vi "Assignment.vi"() -> ()   [LabVIEW 2021]
doc: "https://icons8.com/icon/85465/time\nhttps://icons8.com/icon/44369/cheap-2\nhttps://icons8.com/icon/44372/expensive-price\nhttps://icons8.com/icon/17077/info-squared"
uses:
  Resources/Enum.ctl
  <vilib>/Utility/error.llb/DialogType.ctl
  <vilib>/Utility/file.llb/Write Delimited Spreadsheet (string).vi
panel:
  in  "infoTab":enum32{"InfoTab"}(tab)
  in  "btnInfo":bool
  out "Message":string
  out "isDeluxe":bool
  out "Time Left":dbl(slide) scale=0.0..5.0
  in  "Air Dry \nPosition Switch":bool
  in  "Main Wash \nPosition Switch":bool
  in  "Under Body \nWash Position \nSwitch":bool
  out "Vehicle Out Of Position":bool
  out "Air Dry":bool
  out "Clear Water Rinse":bool
  out "Main High Pressure Wash":bool
  out "Soap Application":bool
  out "Under Body Wash":bool
  in  "btnStop":bool
  in  "btnEconomy":bool
  in  "btnDeluxe":bool
  # "Please select Car Wash Mode"
  # "Deluxe Wash"
  # "Economy Wash"
  # "Message"
  # "Deluxe Wash:\n1. Under Body Wash\n2. Main Car Wash\n3. Air Dry Cycle"
  # "Economy Wash:"
  # "1. Main Car Wash"
  # "approx 25 seconds"
  # "approx 15 seconds"
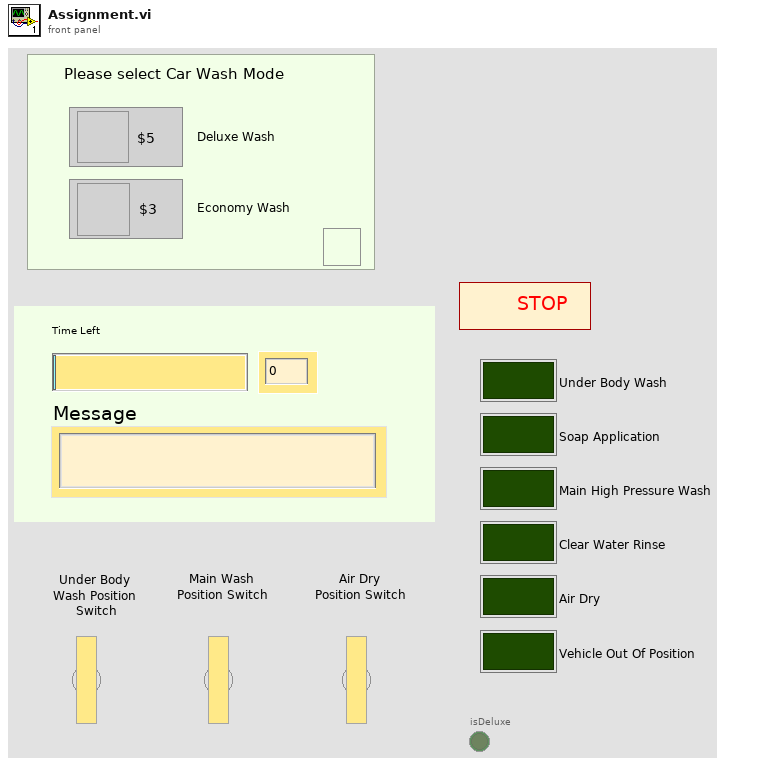
[diagram p1: front panel]
types:
  T1 = typedef "Enum.ctl" = enum16{"Start", "SelectMode", "UnderBodyTimer", "UnderBody", "Soap Timer", "Soap", "MainWashTimer", "MainWash", "RinseTimer", "Rinse", "AirDryTimer", "AirDry", "Trasmit", "End"}
  T2 = enum8{"Enabled", "Disabled", "Disabled and Grayed Out"}
  T3 = typedef "DialogType.ctl" = u16
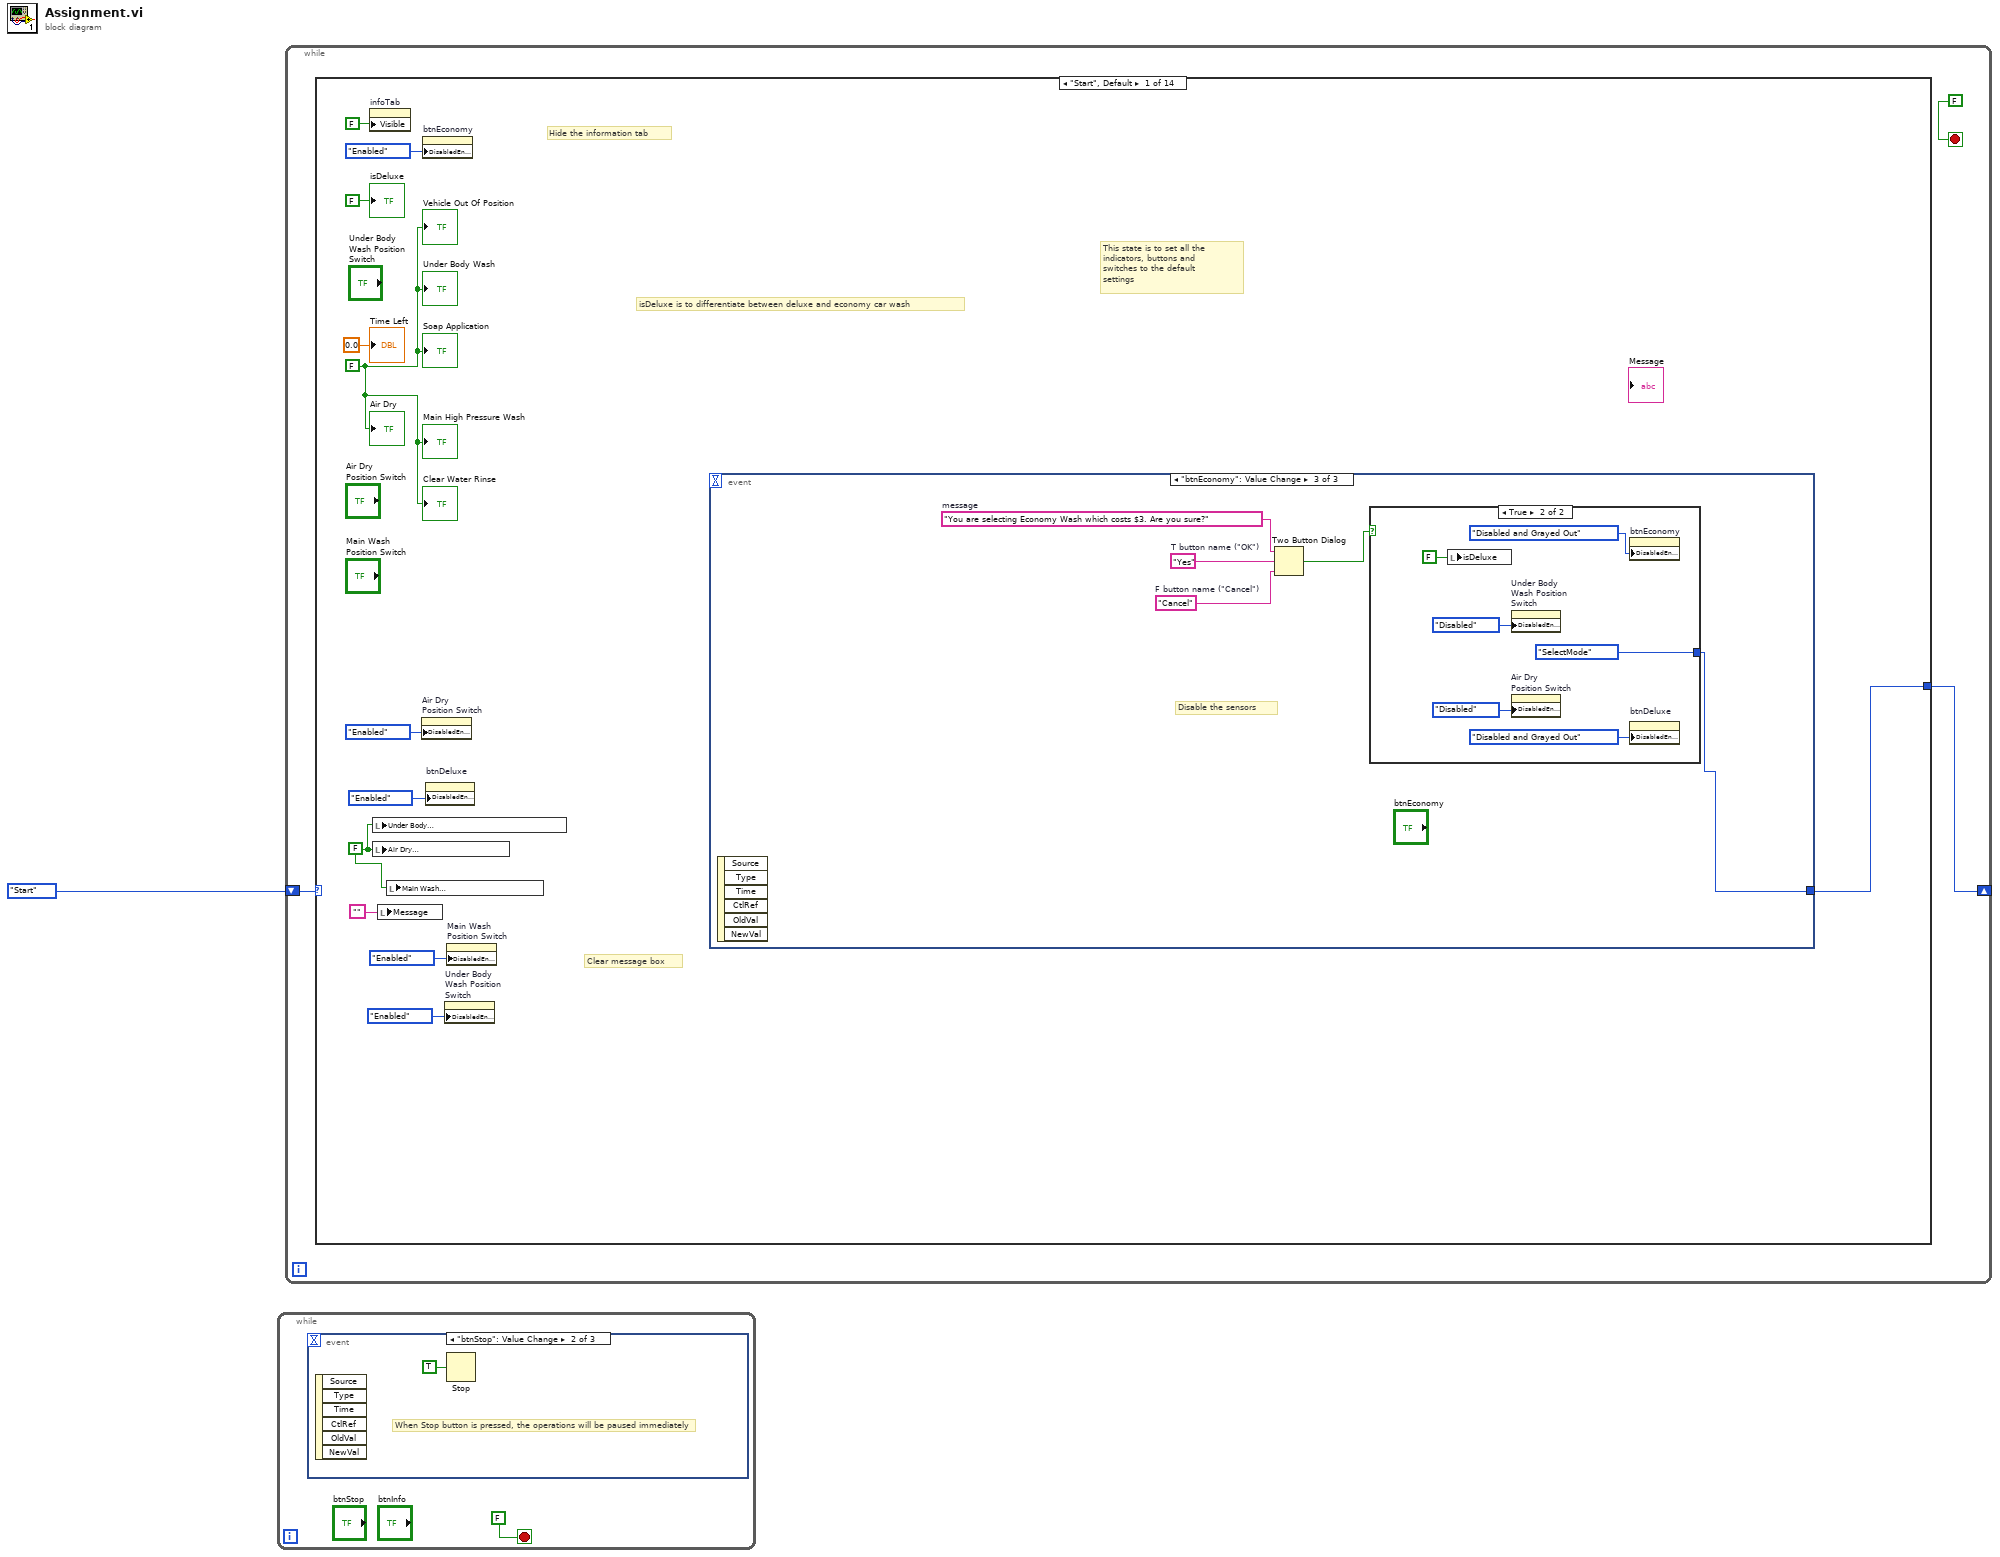
[diagram p0: block diagram]
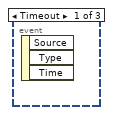
[diagram p2: hidden frame]
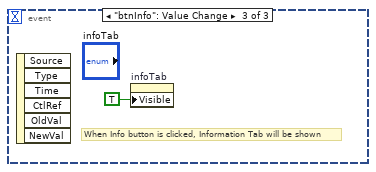
[diagram p3: hidden frame]
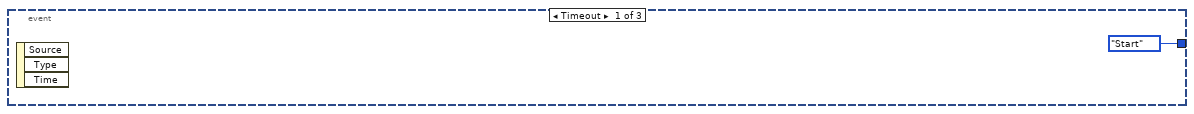
[diagram p4: hidden frame]
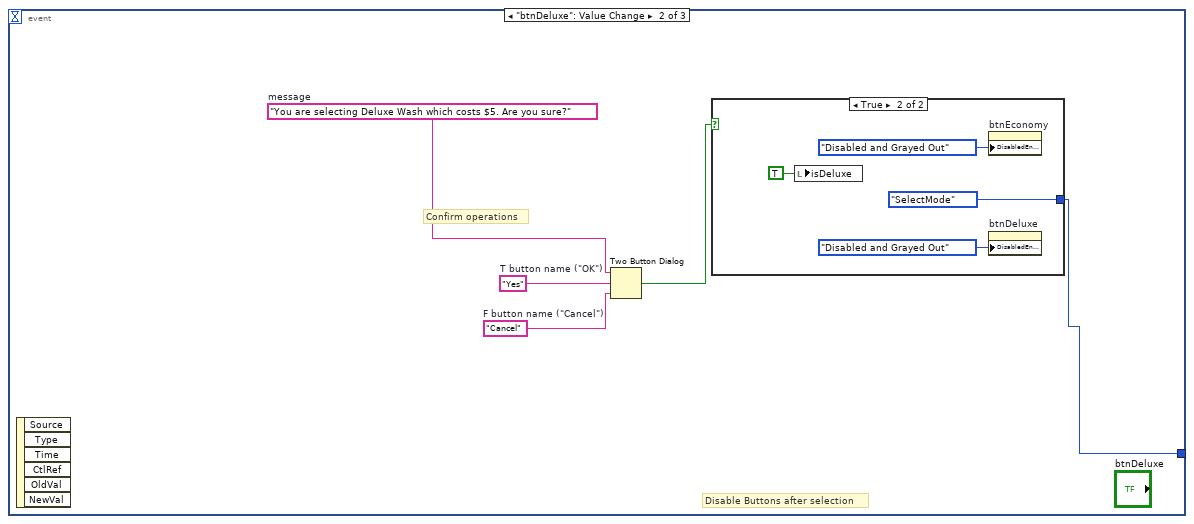
[diagram p5: hidden frame]
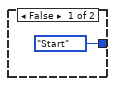
[diagram p6: hidden frame]
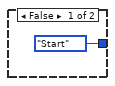
[diagram p7: hidden frame]
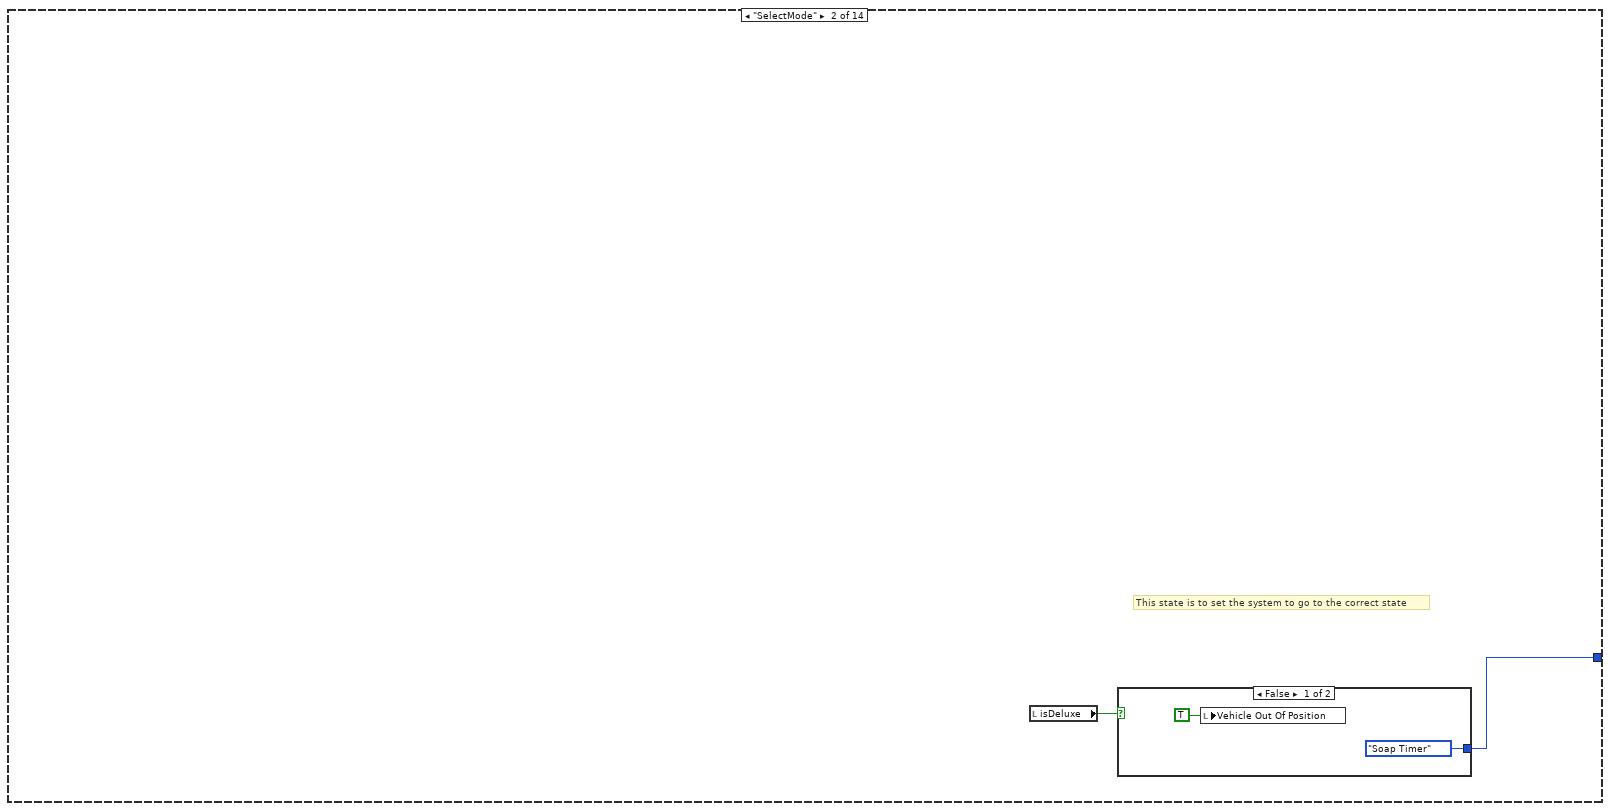
[diagram p8: hidden frame]
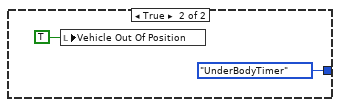
[diagram p9: hidden frame]
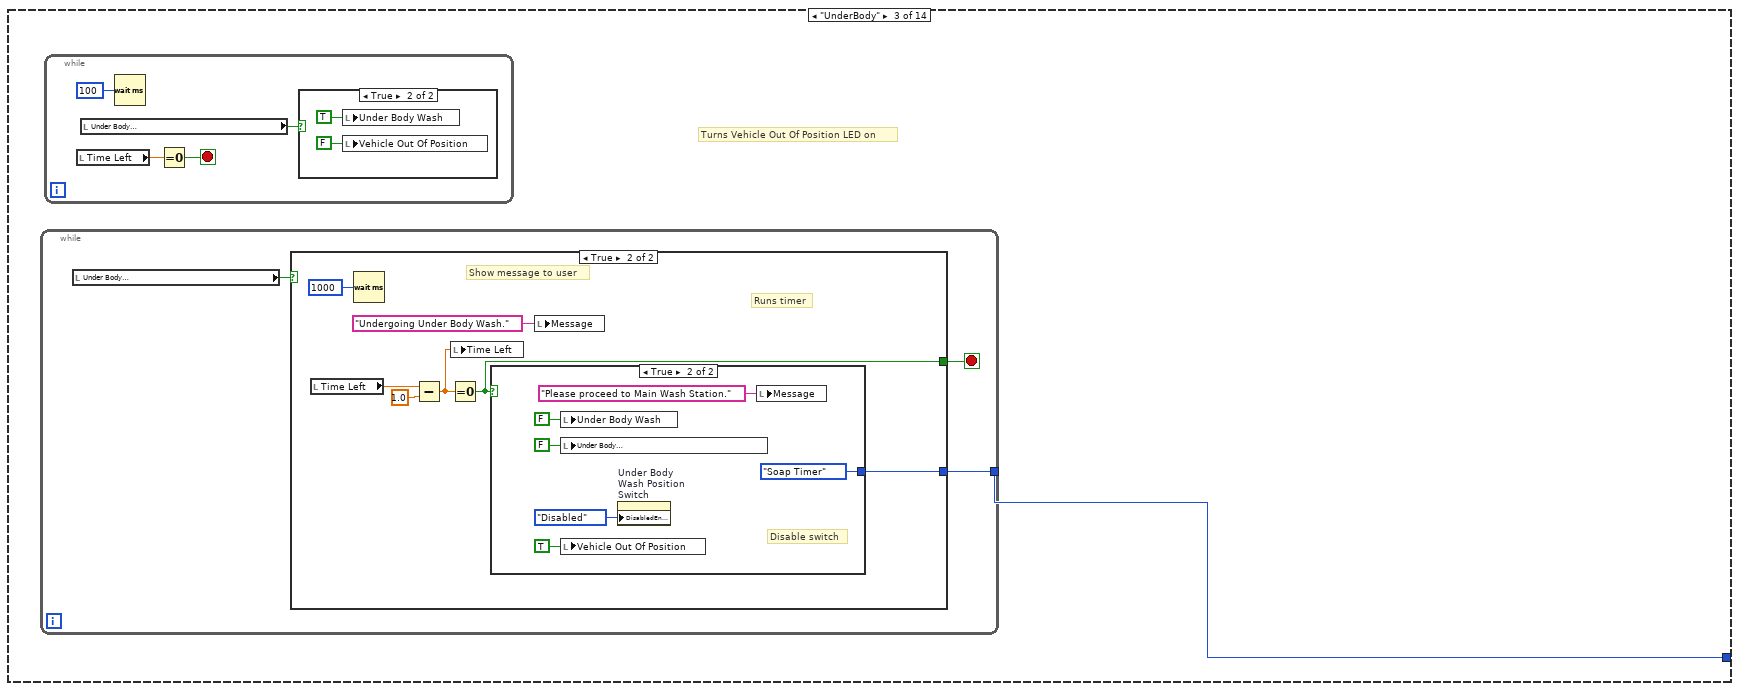
[diagram p10: hidden frame]
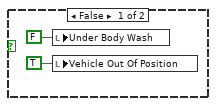
[diagram p11: hidden frame]
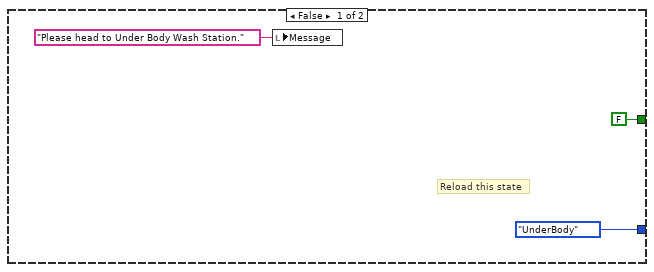
[diagram p12: hidden frame]
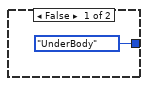
[diagram p13: hidden frame]
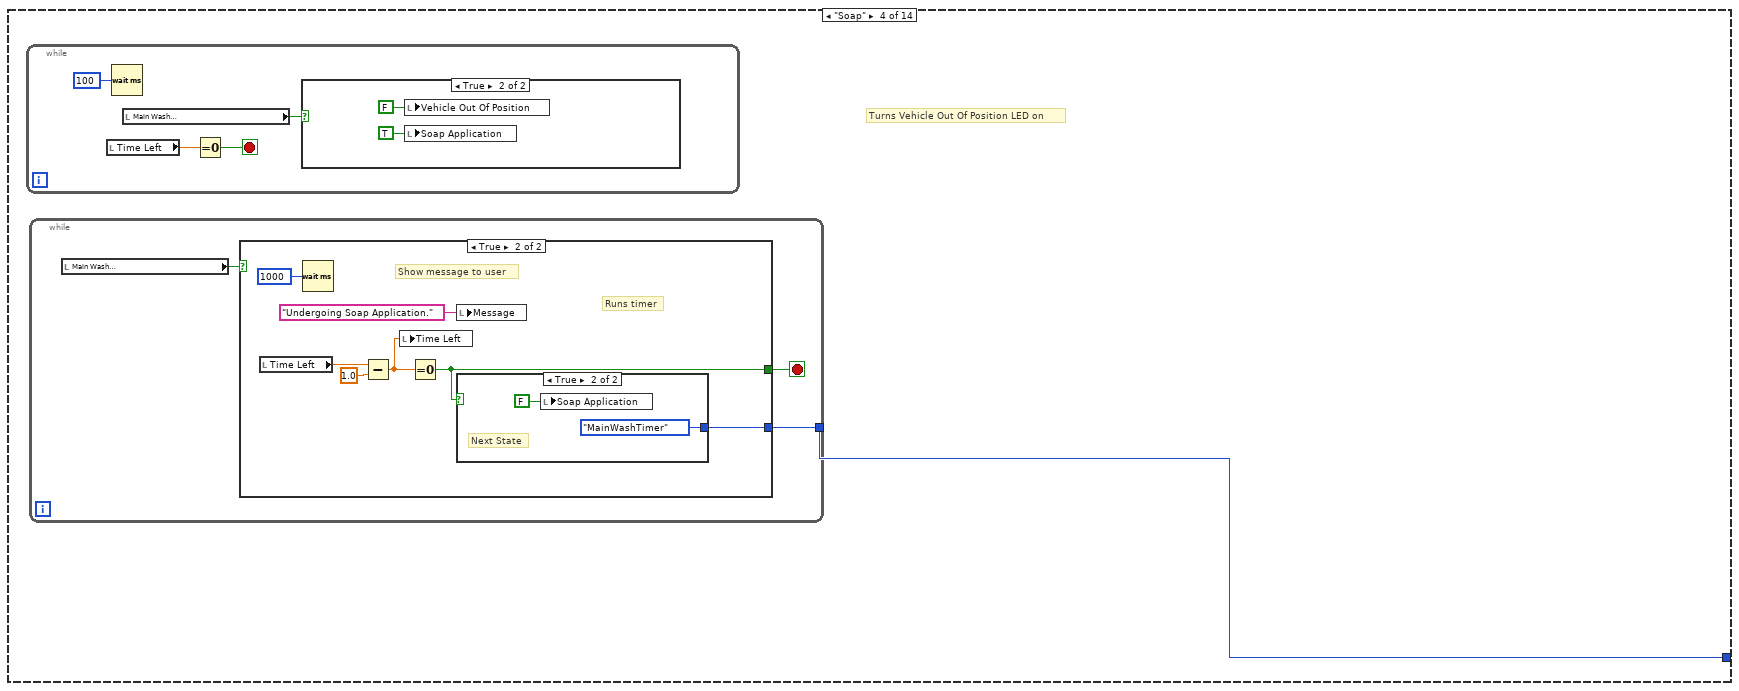
[diagram p14: hidden frame]
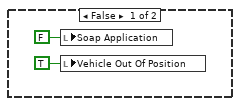
[diagram p15: hidden frame]
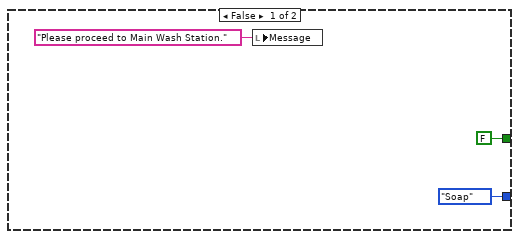
[diagram p16: hidden frame]
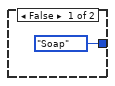
[diagram p17: hidden frame]
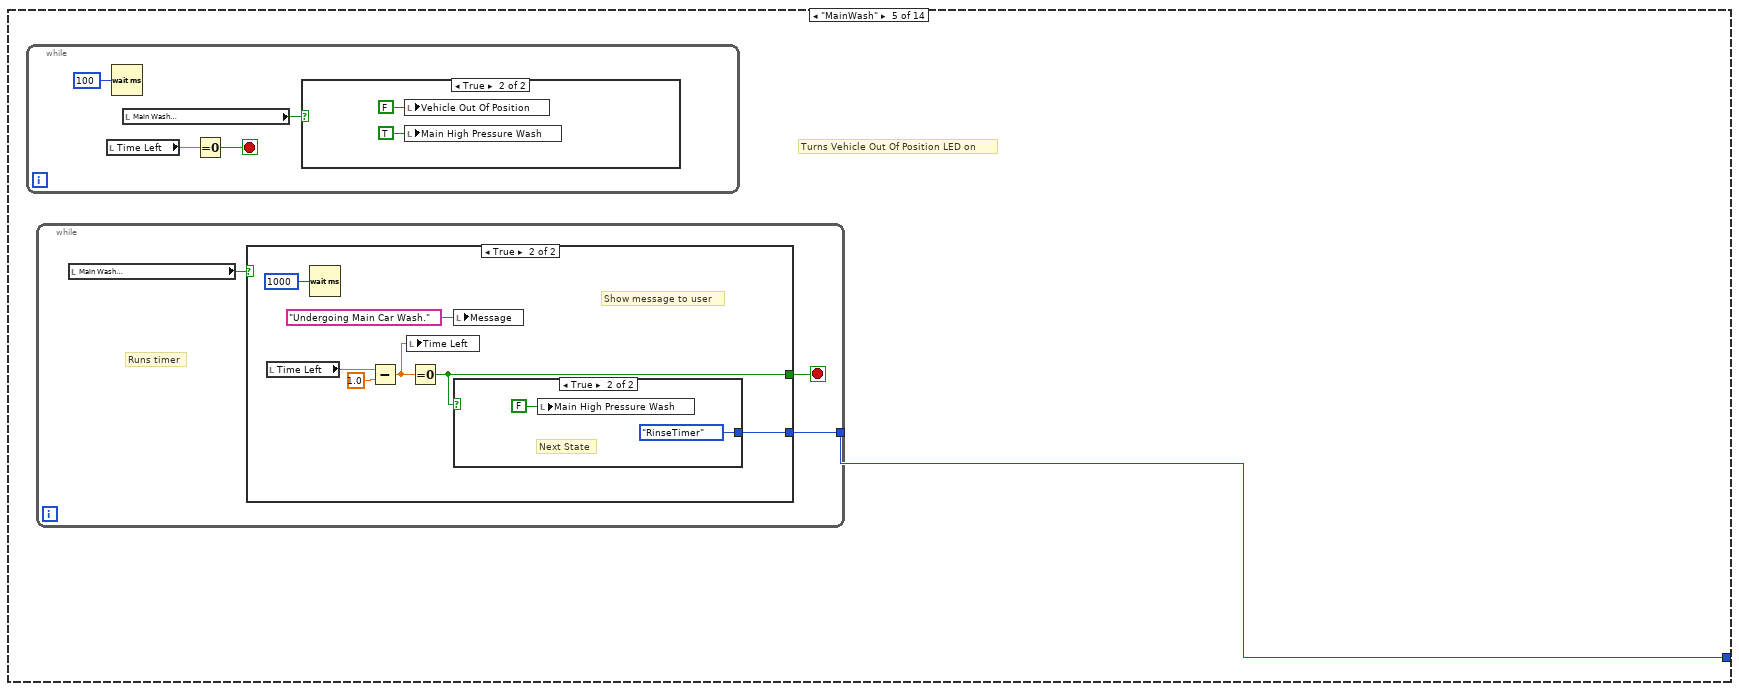
[diagram p18: hidden frame]
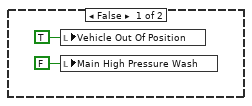
[diagram p19: hidden frame]
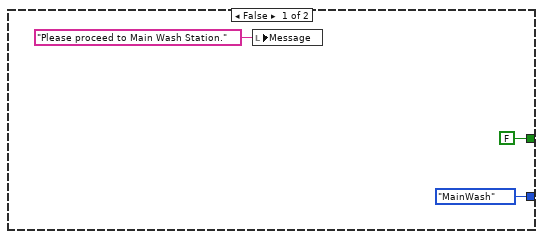
[diagram p20: hidden frame]
diagram:
  n1 = while {
    stop <- FALSE stop-if-true
    n2 = event shown="[1] \"btnStop\": Value Change" {
      selector: _ -> [_ _ _]
      dyn-events: _ -> [_ _ _]
      timeout: _ -> [_ _ _]
      event Timeout {
        n3 = event-data() -> ()  [unwired: 1 in, 3 out]
      }
      event "btnStop": Value Change {
        # "When Stop button is pressed, the operations will be paused immediately"
        n4 = event-data() -> ()  [unwired: 1 in, 6 out]
        n5 = Stop(stop? (T)=TRUE) -> ()
      }
      event "btnInfo": Value Change {
        # "When Info button is clicked, Information Tab will be shown"
        n6 = event-data() -> ()  [unwired: 1 in, 6 out]
        n7 = property on="infoTab" class="TabCtl (strict)"("Visible"=TRUE) -> ()  [unwired: 2 in, 2 out]
      }
    }
  }
  n8 = while {
    shift-right: [w6] -> _
    shift-left: Enum."Start" -> [w7]
    stop <- FALSE stop-if-true
    n9 = case shown="\"Start\", Default" w7 {
      tunnel: [w19 w43 w49 w78 w103 w129 w162 Enum."End" Enum."Start" Enum."UnderBody" Enum."Soap" Enum."MainWash" Enum."Rinse" Enum."AirDry"] -> w6
      frame "Start", Default {
        w8 = FALSE ("Vehicle Out Of Positon")
        w18 = FALSE ("Air Dry \nPosition Switch")
        # "Clear message box"
        # "isDeluxe is to differentiate between deluxe and economy car wash"
        # "Hide the information tab"
        # "This state is to set all the indicators, buttons and switches to the default settings"
        n10 = property on="infoTab" class="TabCtl (strict)"("Visible"=FALSE) -> ()  [unwired: 2 in, 2 out]
        n11 = local write "Under Body \nWash Position \nSwitch"(w18) -> ()
        n12 = local write "Air Dry \nPosition Switch"(w18) -> ()
        n13 = local write "Message"("") -> ()
        n14 = local write "Main Wash \nPosition Switch"(w18) -> ()
        n15 = property on="Air Dry \nPosition Switch" class="Bool (strict)"("DisabledEnum"=T2."Enabled" ("Disabled")) -> ()  [unwired: 2 in, 2 out]
        n16 = property on="btnEconomy" class="Bool"("DisabledEnum"=T2."Enabled" ("Disabled")) -> ()  [unwired: 2 in, 2 out]
        n17 = property on="btnDeluxe" class="Bool"("DisabledEnum"=T2."Enabled" ("Disabled")) -> ()  [unwired: 2 in, 2 out]
        n18 = property on="Under Body \nWash Position \nSwitch" class="Bool (strict)"("DisabledEnum"=T2."Enabled" ("Disabled")) -> ()  [unwired: 2 in, 2 out]
        n19 = property on="Main Wash \nPosition Switch" class="Bool (strict)"("DisabledEnum"=T2."Enabled" ("Disabled")) -> ()  [unwired: 2 in, 2 out]
        n20 = event shown="[2] \"btnEconomy\": Value Change" {
          selector: _ -> [_ _ _]
          dyn-events: _ -> [_ _ _]
          timeout: _ -> [_ _ _]
          tunnel: [Enum."Start" w21 w31] -> w19
          event Timeout {
            n21 = event-data() -> ()  [unwired: 1 in, 3 out]
          }
          event "btnDeluxe": Value Change {
            w23 = "You are selecting Deluxe Wash which costs $5. Are you sure?"  # message
            w24 = "Cancel"  # F button name ("Cancel")
            w25 = "Yes"  # T button name ("OK")
            # "Disable Buttons after selection"
            # "Confirm operations"
            n22 = event-data() -> ()  [unwired: 1 in, 6 out]
            n23 = Two Button Dialog(message=w23, 1:w24, 2:w25) -> (T button?=w22:bool)
            n24 = case shown="True" w22 {
              tunnel: [Enum."Start" ("f") Enum."SelectMode"] -> w21
              frame False {
              }
              frame True {
                n25 = local write "isDeluxe"(TRUE ("isDeluxe")) -> ()
                n26 = property on="btnEconomy" class="Bool"("DisabledEnum"=T2."Disabled and Grayed Out" ("Disabled")) -> ()  [unwired: 2 in, 2 out]
                n27 = property on="btnDeluxe" class="Bool"("DisabledEnum"=T2."Disabled and Grayed Out" ("Disabled")) -> ()  [unwired: 2 in, 2 out]
              }
            }
          }
          event "btnEconomy": Value Change {
            w32 = "You are selecting Economy Wash which costs $3. Are you sure?"  # message
            w34 = "Cancel"  # F button name ("Cancel")
            w33 = "Yes"  # T button name ("OK")
            # "Disable the sensors"
            n28 = event-data() -> ()  [unwired: 1 in, 6 out]
            n29 = Two Button Dialog(message=w32, 1:w34, 2:w33) -> (T button?=w35:bool)
            n30 = case shown="True" w35 {
              tunnel: [Enum."Start" ("f") Enum."SelectMode"] -> w31
              frame False {
              }
              frame True {
                n31 = local write "isDeluxe"(FALSE ("isDeluxe")) -> ()
                n32 = property on="Under Body \nWash Position \nSwitch" class="Bool (strict)"("DisabledEnum"=T2."Disabled" ("Disabled")) -> ()  [unwired: 2 in, 2 out]
                n33 = property on="Air Dry \nPosition Switch" class="Bool (strict)"("DisabledEnum"=T2."Disabled" ("Disabled")) -> ()  [unwired: 2 in, 2 out]
                n34 = property on="btnEconomy" class="Bool"("DisabledEnum"=T2."Disabled and Grayed Out" ("Disabled")) -> ()  [unwired: 2 in, 2 out]
                n35 = property on="btnDeluxe" class="Bool"("DisabledEnum"=T2."Disabled and Grayed Out" ("Disabled")) -> ()  [unwired: 2 in, 2 out]
              }
            }
          }
        }
        "isDeluxe" <- FALSE ("isDeluxe")
        "Time Left" <- 0.0 ("Time Left")
        "Main High Pressure Wash" <- w8
        "Clear Water Rinse" <- w8
        "Air Dry" <- w8
        "Under Body Wash" <- w8
        "Soap Application" <- w8
        "Vehicle Out Of Position" <- w8
      }
      frame "SelectMode" {
        # "This state is to set the system to go to the correct state"
        n36 = local read "isDeluxe"() -> (w44:bool)
        n37 = case shown="False" w44 {
          tunnel: [Enum."Soap Timer" Enum."UnderBodyTimer"] -> w43
          frame False {
            n38 = local write "Vehicle Out Of Position"(TRUE ("Vehicle Out Of Positon")) -> ()
          }
          frame True {
            n39 = local write "Vehicle Out Of Position"(TRUE ("Air Dry")) -> ()
          }
        }
      }
      frame "UnderBody" {
        # "Turns Vehicle Out Of Position LED on"
        n40 = while {
          tunnel: [w60] -> w49
          stop <- w59 stop-if-true
          n41 = local read "Under Body \nWash Position \nSwitch"() -> (w58:bool)
          n42 = case shown="True" w58 {
            tunnel: [Enum."UnderBody" w68] -> w60
            tunnel: [FALSE w65] -> w59
            frame False {
              # "Reload this state"
              n43 = local write "Message"("Please head to Under Body Wash Station.") -> ()
            }
            frame True {
              # "Show message to user"
              # "Runs timer"
              n44 = local read "Time Left"() -> (w69:dbl)
              n45 = Wait (ms)(milliseconds to wait=u32 1000) -> ()  [unwired: 1 out]
              n46 = Subtract(x=w69, y=1.0) -> (x-y=w67:dbl)
              n47 = Equal To 0?(x=w67) -> (x = 0?=w65:bool)
              n48 = local write "Time Left"(w67) -> ()
              n49 = case shown="True" w65 {
                tunnel: [Enum."UnderBody" Enum."Soap Timer"] -> w68
                frame False {
                }
                frame True {
                  # "Disable switch"
                  n50 = local write "Under Body Wash"(FALSE ("Soap Application")) -> ()
                  n51 = local write "Under Body \nWash Position \nSwitch"(FALSE ("Under Body \nWash Position \nSwitch")) -> ()
                  n52 = local write "Vehicle Out Of Position"(TRUE ("Soap Application")) -> ()
                  n53 = property on="Under Body \nWash Position \nSwitch" class="Bool (strict)"("DisabledEnum"=T2."Disabled" ("Disabled")) -> ()  [unwired: 2 in, 2 out]
                  n54 = local write "Message"("Please proceed to Main Wash Station." ("Station")) -> ()
                }
              }
              n55 = local write "Message"("Undergoing Under Body Wash." ("Station")) -> ()
            }
          }
        }
        n56 = while {
          stop <- w50 stop-if-true
          n57 = local read "Time Left"() -> (w51:dbl)
          n58 = local read "Under Body \nWash Position \nSwitch"() -> (w52:bool)
          n59 = Wait (ms)(milliseconds to wait=u32 100) -> ()  [unwired: 1 out]
          n60 = Equal To 0?(x=w51) -> (x = 0?=w50:bool)
          n61 = case shown="True" w52 {
            frame False {
              n62 = local write "Under Body Wash"(FALSE ("Soap Application")) -> ()
              n63 = local write "Vehicle Out Of Position"(TRUE ("Soap Application")) -> ()
            }
            frame True {
              n64 = local write "Under Body Wash"(TRUE ("Soap Application")) -> ()
              n65 = local write "Vehicle Out Of Position"(FALSE ("Vehicle Out Of Positon")) -> ()
            }
          }
        }
      }
      frame "Soap" {
        # "Turns Vehicle Out Of Position LED on"
        n66 = while {
          stop <- w79 stop-if-true
          n67 = local read "Time Left"() -> (w80:dbl)
          n68 = Wait (ms)(milliseconds to wait=u32 100) -> ()  [unwired: 1 out]
          n69 = local read "Main Wash \nPosition Switch"() -> (w82:bool)
          n70 = Equal To 0?(x=w80) -> (x = 0?=w79:bool)
          n71 = case shown="True" w82 {
            frame False {
              n72 = local write "Soap Application"(FALSE ("Soap Application")) -> ()
              n73 = local write "Vehicle Out Of Position"(TRUE ("Soap Application")) -> ()
            }
            frame True {
              n74 = local write "Vehicle Out Of Position"(FALSE ("Vehicle Out Of Positon")) -> ()
              n75 = local write "Soap Application"(TRUE ("Soap Application")) -> ()
            }
          }
        }
        n76 = while {
          tunnel: [w88] -> w78
          stop <- w89 stop-if-true
          n77 = local read "Main Wash \nPosition Switch"() -> (w87:bool)
          n78 = case shown="True" w87 {
            tunnel: [Enum."Soap" w98] -> w88
            tunnel: [FALSE w95] -> w89
            frame False {
              n79 = local write "Message"("Please proceed to Main Wash Station.") -> ()
            }
            frame True {
              # "Show message to user"
              # "Runs timer"
              n80 = local read "Time Left"() -> (w99:dbl)
              n81 = Wait (ms)(milliseconds to wait=u32 1000) -> ()  [unwired: 1 out]
              n82 = Subtract(x=w99, y=1.0) -> (x-y=w97:dbl)
              n83 = local write "Time Left"(w97) -> ()
              n84 = Equal To 0?(x=w97) -> (x = 0?=w95:bool)
              n85 = local write "Message"("Undergoing Soap Application." ("Station")) -> ()
              n86 = case shown="True" w95 {
                tunnel: [Enum."Soap" Enum."MainWashTimer"] -> w98
                frame False {
                }
                frame True {
                  # "Next State"
                  n87 = local write "Soap Application"(FALSE ("Soap Application")) -> ()
                }
              }
            }
          }
        }
      }
      frame "MainWash" {
        # "Turns Vehicle Out Of Position LED on"
        n88 = while {
          stop <- w104 stop-if-true
          n89 = local read "Time Left"() -> (w105:dbl)
          n90 = Wait (ms)(milliseconds to wait=u32 100) -> ()  [unwired: 1 out]
          n91 = local read "Main Wash \nPosition Switch"() -> (w107:bool)
          n92 = Equal To 0?(x=w105) -> (x = 0?=w104:bool)
          n93 = case shown="True" w107 {
            frame False {
              n94 = local write "Vehicle Out Of Position"(TRUE ("Soap Application")) -> ()
              n95 = local write "Main High Pressure Wash"(FALSE ("Soap Application")) -> ()
            }
            frame True {
              n96 = local write "Vehicle Out Of Position"(FALSE ("Vehicle Out Of Positon")) -> ()
              n97 = local write "Main High Pressure Wash"(TRUE ("Soap Application")) -> ()
            }
          }
        }
        n98 = while {
          tunnel: [w114] -> w103
          stop <- w112 stop-if-true
          # "Runs timer"
          n99 = local read "Main Wash \nPosition Switch"() -> (w113:bool)
          n100 = case shown="True" w113 {
            tunnel: [Enum."MainWash" w123] -> w114
            tunnel: [FALSE w120] -> w112
            frame False {
              n101 = local write "Message"("Please proceed to Main Wash Station.") -> ()
            }
            frame True {
              # "Show message to user"
              n102 = local read "Time Left"() -> (w124:dbl)
              n103 = Wait (ms)(milliseconds to wait=u32 1000) -> ()  [unwired: 1 out]
              n104 = Subtract(x=w124, y=1.0) -> (x-y=w122:dbl)
              n105 = local write "Time Left"(w122) -> ()
              n106 = Equal To 0?(x=w122) -> (x = 0?=w120:bool)
              n107 = local write "Message"("Undergoing Main Car Wash." ("Station")) -> ()
              n108 = case shown="True" w120 {
                tunnel: [Enum."MainWash" Enum."RinseTimer"] -> w123
                frame False {
                  n109 = Wait (ms)(milliseconds to wait=u32 1000) -> ()  [unwired: 1 out]
                }
                frame True {
                  # "Next State"
                  n110 = local write "Main High Pressure Wash"(FALSE ("Soap Application")) -> ()
                }
              }
            }
          }
        }
      }
      frame "Rinse" {
        # "Turns Vehicle Out Of Position LED on"
        n111 = while {
          stop <- w130 stop-if-true
          n112 = local read "Time Left"() -> (w131:dbl)
          n113 = Wait (ms)(milliseconds to wait=u32 100) -> ()  [unwired: 1 out]
          n114 = local read "Main Wash \nPosition Switch"() -> (w133:bool)
          n115 = Equal To 0?(x=w131) -> (x = 0?=w130:bool)
          n116 = case shown="False" w133 {
            frame False {
              n117 = local write "Clear Water Rinse"(FALSE ("Soap Application")) -> ()
              n118 = local write "Vehicle Out Of Position"(TRUE ("Soap Application")) -> ()
            }
            frame True {
              n119 = local write "Clear Water Rinse"(TRUE ("Soap Application")) -> ()
              n120 = local write "Vehicle Out Of Position"(FALSE ("Vehicle Out Of Positon")) -> ()
            }
          }
        }
        n121 = while {
          tunnel: [w140] -> w129
          stop <- w138 stop-if-true
          # "Runs timer"
          n122 = local read "Main Wash \nPosition Switch"() -> (w139:bool)
          n123 = case shown="True" w139 {
            tunnel: [Enum."Rinse" w149] -> w140
            tunnel: [FALSE w146] -> w138
            frame False {
              n124 = local write "Message"("Please proceed to Main Wash Station.") -> ()
            }
            frame True {
              # "Show message to user"
              n125 = local read "Time Left"() -> (w150:dbl)
              n126 = Wait (ms)(milliseconds to wait=u32 1000) -> ()  [unwired: 1 out]
              n127 = Subtract(x=w150, y=1.0) -> (x-y=w148:dbl)
              n128 = Equal To 0?(x=w148) -> (x = 0?=w146:bool)
              n129 = local write "Time Left"(w148) -> ()
              n130 = case shown="True" w146 {
                tunnel: [Enum."Rinse" w154] -> w149
                frame False {
                }
                frame True {
                  n131 = local read "isDeluxe"() -> (w155:bool)
                  n132 = local write "Main Wash \nPosition Switch"(FALSE ("Main Wash \nPosition Switch")) -> ()
                  n133 = local write "Clear Water Rinse"(FALSE ("Soap Application")) -> ()
                  n134 = case shown="True" w155 {
                    tunnel: [Enum."Trasmit" Enum."AirDryTimer"] -> w154
                    frame False {
                      n135 = property on="Air Dry \nPosition Switch" class="Bool (strict)"("DisabledEnum"=T2."Disabled" ("Disabled")) -> ()  [unwired: 2 in, 2 out]
                      n136 = local write "Message"("Car Wash Operation Completed." ("Station")) -> ()
                    }
                    frame True {
                      # "Next State"
                      n137 = local write "Message"("Kindly proceed to Air Dry Station." ("Station")) -> ()
                    }
                  }
                  n138 = property on="Main Wash \nPosition Switch" class="Bool (strict)"("DisabledEnum"=T2."Disabled" ("Disabled")) -> ()  [unwired: 2 in, 2 out]
                }
              }
              n139 = local write "Message"("Undergoing Clear Water Rinse." ("Station")) -> ()
            }
          }
        }
      }
      frame "AirDry" {
        # "Turns Vehicle Out Of Position LED on"
        n140 = while {
          stop <- w163 stop-if-true
          n141 = local read "Time Left"() -> (w164:dbl)
          n142 = local read "Air Dry \nPosition Switch"() -> (w166:bool)
          n143 = Wait (ms)(milliseconds to wait=u32 100) -> ()  [unwired: 1 out]
          n144 = Equal To 0?(x=w164) -> (x = 0?=w163:bool)
          n145 = case shown="False" w166 {
            frame False {
              n146 = local write "Air Dry"(FALSE ("Soap Application")) -> ()
              n147 = local write "Vehicle Out Of Position"(TRUE ("Soap Application")) -> ()
            }
            frame True {
              n148 = local write "Air Dry"(TRUE ("Soap Application")) -> ()
              n149 = local write "Vehicle Out Of Position"(FALSE ("Vehicle Out Of Positon")) -> ()
            }
          }
        }
        n150 = while {
          tunnel: [w173] -> w162
          stop <- w172 stop-if-true
          # "Runs timer"
          n151 = local read "Air Dry \nPosition Switch"() -> (w171:bool)
          n152 = case shown="True" w171 {
            tunnel: [Enum."AirDry" w181] -> w173
            tunnel: [FALSE w178] -> w172
            frame False {
              n153 = local write "Message"("Kindly proceed to Air Dry Station." ("Station")) -> ()
            }
            frame True {
              # "Show message to user"
              n154 = local read "Time Left"() -> (w182:dbl)
              n155 = Wait (ms)(milliseconds to wait=u32 1000) -> ()  [unwired: 1 out]
              n156 = Subtract(x=w182, y=1.0) -> (x-y=w180:dbl)
              n157 = Equal To 0?(x=w180) -> (x = 0?=w178:bool)
              n158 = local write "Time Left"(w180) -> ()
              n159 = local write "Message"("Undergoing Air Dry Cycle." ("Station")) -> ()
              n160 = case shown="True" w178 {
                tunnel: [Enum."AirDry" Enum."Trasmit"] -> w181
                frame False {
                }
                frame True {
                  # "Disable switch"
                  # "Next State"
                  n161 = local write "Air Dry"(FALSE ("Soap Application")) -> ()
                  n162 = property on="Air Dry \nPosition Switch" class="Bool (strict)"("DisabledEnum"=T2."Disabled" ("Disabled")) -> ()  [unwired: 2 in, 2 out]
                  n163 = local write "Message"("Car Wash Operation Completed." ("Station")) -> ()
                }
              }
            }
          }
        }
      }
      frame "Trasmit" {
        w190 = T3 0 items=["no dialog", "OK message", "continue or stop message", "OK message + warnings", "continue/stop + warnings"] ("type of dialog (OK msg:1)")
        w193 = 1  # dimension size
        # "Save Errors"
        # "Reshape 1D array to 2D"
        # "Change numeric code to String"
        # "TypeOfWash"
        # "Time String"
        # "Date String"
        n164 = Format Date/Time String(time format string (%c)="%d/%m/%Y") -> (date/time string=w198:string)  [unwired: 2 in]
        n165 = TCP Open Connection(remote port or service name=u16 1234, timeout ms (60000)=60000) -> (connection ID=w215:refnum<k5>, error out=w214:errorcluster)  [unwired: 3 in]
        n166 = local read "isDeluxe"() -> (w216:bool)
        n167 = Format Date/Time String(time format string (%c)="%I:%M %p") -> (date/time string=w197:string)  [unwired: 2 in]
        n168 = case shown="True" w216 {
          tunnel: ["Economy" "Deluxe"] -> w207
          frame False {
          }
          frame True {
          }
        }
        n169 = TCP Write(connection ID=w215, data in=w198, error in (no error)=w214) -> (connection ID out=w212:refnum<k5>, error out=w213:errorcluster)  [unwired: 1 in, 1 out]
        n170 = TCP Write(connection ID=w212, data in=w197, error in (no error)=w213) -> (connection ID out=w211:refnum<k5>, error out=w210:errorcluster)  [unwired: 1 in, 1 out]
        n171 = TCP Write(connection ID=w211, data in=w207, error in (no error)=w210) -> (connection ID out=w209:refnum<k5>, error out=w208:errorcluster)  [unwired: 1 in, 1 out]
        n172 = TCP Close Connection(connection ID=w209, error in (no error)=w208) -> (error out=w204:errorcluster)  [unwired: 1 in, 1 out]
        n173 = call <vilib>:"Simple Error Handler.vi"("type of dialog (OK msg:1)"=w190, "error in (no error)"=w204) -> ("code out"=w196:i32, "source out"=w189:string)  [unwired: 3 in, 3 out]
        n174 = Number To Decimal String(number=w196) -> (decimal integer string=w195:string)  [unwired: 1 in]
        n175 = Build Array "Build Array"(w198, w197, w195, w189) -> (w194:string[])
        n176 = call <vilib>:"Application Directory.vi"() -> ("Application Directory"=w203:path)
        n177 = Reshape Array "Reshape Array"(w194, w193, 4 ("dimension size")) -> (w191:string[][])
        n178 = Build Path(base path=w203, name or relative path=path "Resources/ErrorList.csv") -> (appended path=w201:path)
        n179 = call-poly <vilib>:"Write Delimited Spreadsheet.vi"("file path (dialog if empty)"=w201, "2D data"=w191, "append to file? (new file:F)"=TRUE, "delimiter (\\t)"="," ("delimiter (\\t)")) -> ()  [unwired: 10 in, 2 out]
      }
      frame "End" {
        # "Inform user that the operation is completed"
        n180 = One Button Dialog(message="Automated Wash is done and is recorded into the system. ") -> ()  [unwired: 1 in, 1 out]
      }
      frame "UnderBodyTimer" {
        # "Set Scale of slider"
        # "Set Timer for Each Cycle"
        n181 = local write "Time Left"(10.0 ("Time Left")) -> ()
        n182 = property on="Time Left" class="Slide (strict)"("Scale.Maximum"=10.0 ("Scale.Range:Maximum")) -> ()  [unwired: 2 in, 2 out]
      }
      frame "Soap Timer" {
        # "Set Scale of slider"
        # "Set Timer for Each Cycle"
        n183 = local write "Time Left"(5.0 ("Time Left")) -> ()
        n184 = property on="Time Left" class="Slide (strict)"("Scale.Maximum"=5.0 ("Scale.Range:Maximum")) -> ()  [unwired: 2 in, 2 out]
      }
      frame "MainWashTimer" {
        # "Set Timer for Each Cycle"
        n185 = local write "Time Left"(5.0 ("Time Left")) -> ()
        n186 = local write "Soap Application"(FALSE ("Soap Application")) -> ()
      }
      frame "RinseTimer" {
        # "Set Timer for Each Cycle"
        n187 = local write "Time Left"(5.0 ("Time Left")) -> ()
        n188 = local write "Main High Pressure Wash"(FALSE ("Soap Application")) -> ()
      }
      frame "AirDryTimer" {
        # "Set Timer for Each Cycle"
        # "Set Scale of slider"
        n189 = local write "Time Left"(10.0 ("Time Left")) -> ()
        n190 = property on="Time Left" class="Slide (strict)"("Scale.Maximum"=10.0 ("Scale.Range:Maximum")) -> ()  [unwired: 2 in, 2 out]
      }
    }
  }
